vi "Launcher_JKI.vi"() -> ()   [LabVIEW 2022 SP3]
uses:
  XY Stage/Axis Objects/iMotion Controller/iMotion Controller.lvclass
  148c7043-a0e6-40f1-af8e-846f2eb82a0e.vi
  58421ff6-31ce-4a07-9265-554c6ce1187d.vi
  148c7043-a0e6-40f1-af8e-846f2eb82a0e.vi/a9559f68-c05e-40f8-8ef8-fb73dbc3861a.vi
  58421ff6-31ce-4a07-9265-554c6ce1187d.vi/a9559f68-c05e-40f8-8ef8-fb73dbc3861a.vi
  XY Stage/JKI State Machine/Syncronus/Sync 2-Axis Stage Controller.lvclass
  C:/Stage-Work/XY Stage/JKI State Machine/Syncronus 2-Axis Stage/Syncronus 2-Axis Stage.lvclass
  <vilib>/Utility/LVClass/Get LV Class Default Value.vi
  XY Stage/Framework/Read Configs/Read Configs Sections.lvlib
  XY Stage/JKI State Machine/UI/JKI UI.lvlib
panel:
  out "error out":errorcluster
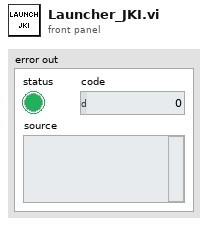
[diagram p1: front panel]
types:
  T1 = typedef "Read Configs Sections.lvlib/Section Data.ctl" = cluster{"Path":path, "Section":string}
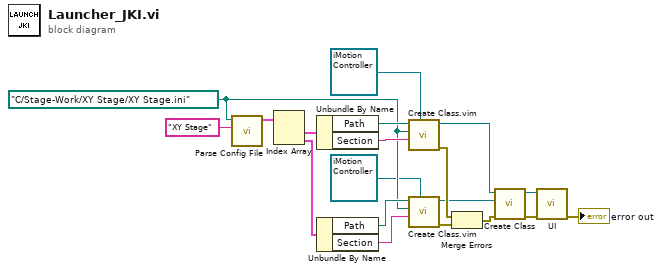
[diagram p0: block diagram]
diagram:
  w6 = path "C:/Stage-Work/XY Stage/XY Stage.ini" ("Config Path")
  n1 = call "Parse Config File.vi"("Section"="XY Stage", "Config Path"=w6) -> ("Array"=w19:T1[])  [unwired: 8 in, 1 out]
  n2 = Index Array(array=w19) -> (element #1=w18:T1, element #2=w17:T1)  [unwired: 2 in]
  n3 = Unbundle By Name(w18) -> ("Path"=w9:path, "Section"=w8:string)
  n4 = Unbundle By Name(w17) -> ("Path"=w7:path, "Section"=w3:string)
  n5 = call "Create Class.vim"("Dynamic Load.lvclass"=refnum<class "iMotion Controller.lvclass"> refnum ("iMotion Controller.lvclass"), "Section"=w8, "Config Path"=w6, "Class Path"=w9) -> ("error out"=w15:errorcluster, "Dynamic Load out"=w13:refnum<class "iMotion Controller.lvclass">)  [unwired: 6 in]
  n6 = call "Create Class.vim"("Dynamic Load.lvclass"=refnum<class "iMotion Controller.lvclass"> refnum ("iMotion Controller.lvclass"), "Section"=w3, "Config Path"=w6, "Class Path"=w7) -> ("error out"=w14:errorcluster, "Dynamic Load out"=w12:refnum<class "iMotion Controller.lvclass">)  [unwired: 6 in]
  n7 = Merge Errors(w15, w14) -> (w11:errorcluster)
  n8 = call "Create Class.vi"("error in (no error)"=w11, "Y-Axis"=w12, "X-Axis"=w13) -> ("error out"=w1:errorcluster, "Sync 2-Axis Stage Controller out"=w2:refnum<class "Sync 2-Axis Stage Controller.lvclass">)  [unwired: 7 in]
  n9 = call "UI.vi"("error"=w1, "2-axis"=w2) -> ("error out"=→"error out":errorcluster)  [unwired: 9 in]
